vi "Collect Data.vi"(0 "Location of FieldMax2Lib.dll in":path=path "C:/Windows/SysWOW64/FieldMax2Lib.dll", 1 "Meter ID in":i32) -> (7 "Location of FieldMax2Lib.dll out":path, 8 "Meter ID out":i32, 9 "Measurement":sgl, 10 "Period":u32)   [LabVIEW 2018]
panel:
  # "This VI is used to collect streaming measurement data from the meter's buffer.\n\nIf the Measurement data appears to not be matching up with the data on the meter's display, doing a Re-Sync should clear the meter's buffer and synchronize the readings again.\n\nThe Period value is only used with energy measurements and can be converted to the rep rate at which pulses are being collected by the meter.\n1 / (Period x 8 usec) = Rep Rate"
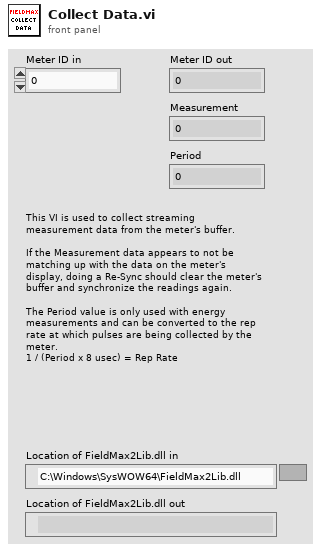
[diagram p1: front panel]
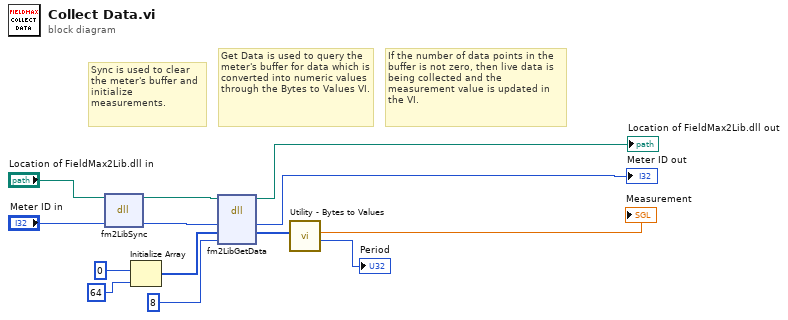
[diagram p0: block diagram]
diagram:
  # "If the number of data points in the buffer is not zero, then live data is being collected and the measurement value is updated in the VI."
  # "Get Data is used to query the meter's buffer for data which is converted into numeric values through the Bytes to Values VI."
  # "Sync is used to clear the meter's buffer and initialize measurements."
  n1 = dll-call lib="C:/Windows/System32/FieldMax2Lib.dll" fn="fm2LibSync" label="Sync"(path in="Location of FieldMax2Lib.dll in", "h"="Meter ID in") -> (path out=w5:path, "h"=w4:i32)  [unwired: 3 in, 1 out]
  n2 = Initialize Array(u8 0 ("element"), 64 ("dimension size")) -> (w11:u8[])
  n3 = dll-call lib="C:/Windows/System32/FieldMax2Lib.dll" fn="fm2LibGetData" label="Get Data"(path in=w5, "h"=w4, "returnBuffer"=w11, "count"=i16 8) -> (path out=→"Location of FieldMax2Lib.dll out":path, "h"=→"Meter ID out":i32, "returnBuffer"=w2:u8[])  [unwired: 4 in, 1 out]
  n4 = call "Utility - Bytes to Values.vi"("DataBuffer"=w2) -> ("Period"=→"Period":u32, "Measurement Value"=→"Measurement":sgl)  [unwired: 9 in]
